vi "SOL Instruments LS.vi"() -> ()   [LabVIEW 2015]
doc: "Example VI that demonstrates all library features."
uses:
  PL SOL Instruments MS.lvclass
panel:
  in  "slit configuration":cluster{"width, um":dbl, "reset":bool}
  in  "slit":u8(ring)
  in  "mirror position index":u8(ring)
  in  "mirror":u8(ring)
  in  "shutter state":bool
  in  "shutter":u8(ring) items=["Shutter S1"]
  in  "turret configuration":T1 {"grating" items=["1200; 750", "1200; 280"]}
  in  "turret":u8(ring) items=["Change of the gratings"]
  in  "configuration file path":path
  out "SOL MS":refnum<class "PL SOL Instruments MS.lvclass">
  in  "port":refnum<visa-resource-name>
  out "error":errorcluster
  in  "stop":bool
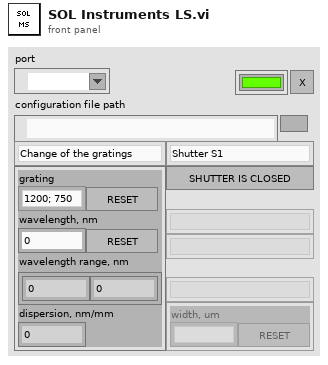
[diagram p1: front panel]
types:
  T1 = cluster{"grating":u8, "reset grating":bool, "wavelength, nm":dbl, "reset wavelength":bool, "wavelength range, nm":cluster{"min":dbl, "max":dbl}, "dispersion, nm/mm":dbl}
  T2 = cluster{"turrets":cluster{"name":string, "gratings":cluster{"name":string, "groove density, g/mm":dbl, "blaze wavelength, nm":dbl, "min wavelength, nm":dbl, "max wavelength, nm":dbl}[]}[], "shutters":cluster{"name":string}[], "mirrors":cluster{"name":string, "positions":cluster{"name":string}[]}[], "slits":cluster{"name":string, "min width, um":dbl, "max width, um":dbl}[]}
  T3 = cluster{"turrets":cluster{"current grating index":u8, "wavelength, nm":dbl, "dispersion, nm/mm":dbl}[], "shutters":cluster{"is open":bool}[], "mirrors":cluster{"current position index":u8}[], "slits":cluster{"width, um":dbl}[]}
  T4 = cluster{"name":string, "gratings":cluster{"name":string, "groove density, g/mm":dbl, "blaze wavelength, nm":dbl, "min wavelength, nm":dbl, "max wavelength, nm":dbl}[]}[]
  T5 = cluster{"current grating index":u8, "wavelength, nm":dbl, "dispersion, nm/mm":dbl}[]
  T6 = cluster{"name":string, "gratings":cluster{"name":string, "groove density, g/mm":dbl, "blaze wavelength, nm":dbl, "min wavelength, nm":dbl, "max wavelength, nm":dbl}[]}
  T7 = cluster{"current grating index":u8, "wavelength, nm":dbl, "dispersion, nm/mm":dbl}
  T8 = cluster{"name":string, "groove density, g/mm":dbl, "blaze wavelength, nm":dbl, "min wavelength, nm":dbl, "max wavelength, nm":dbl}[]
  T9 = cluster{"name":string, "groove density, g/mm":dbl, "blaze wavelength, nm":dbl, "min wavelength, nm":dbl, "max wavelength, nm":dbl}
  T10 = enum8{"Enabled", "Disabled", "Disabled and Grayed Out"}
  T11 = cluster{"name":string, "positions":cluster{"name":string}[]}[]
  T12 = cluster{"name":string, "min width, um":dbl, "max width, um":dbl}[]
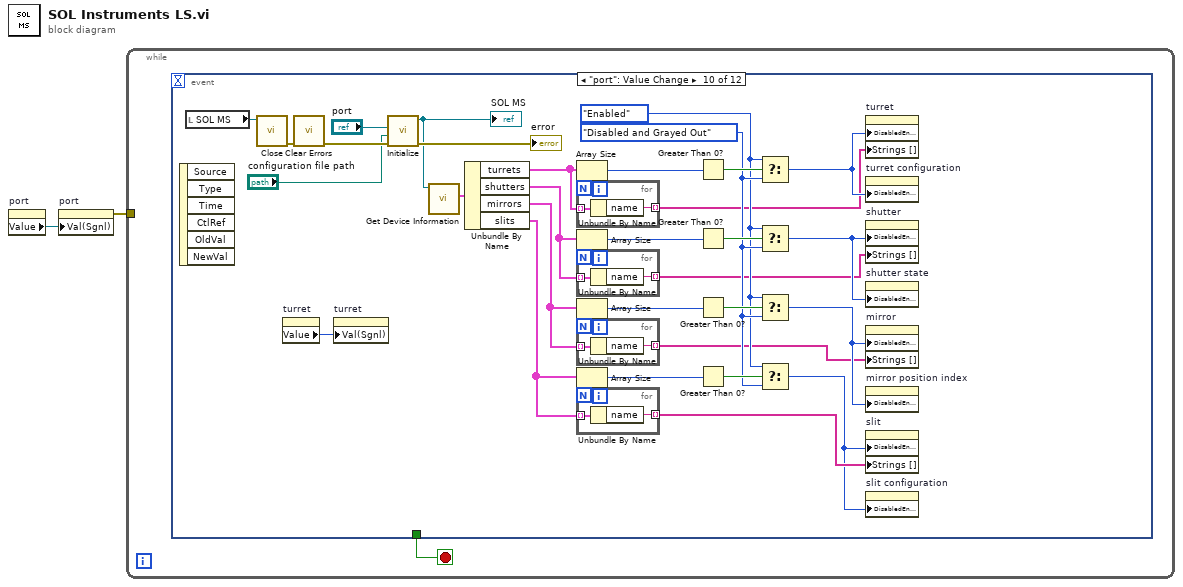
[diagram p0: block diagram]
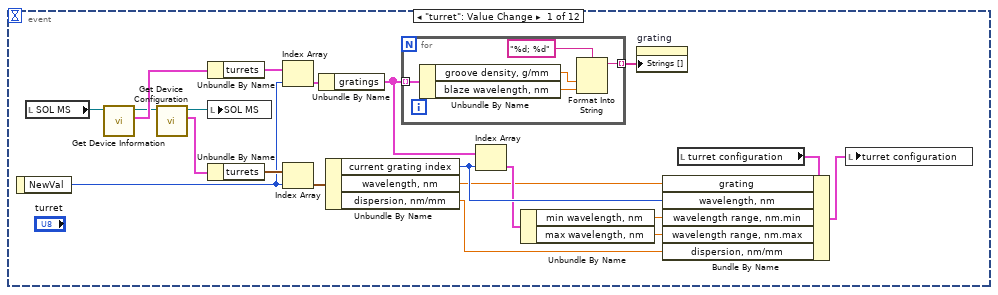
[diagram p2: hidden frame]
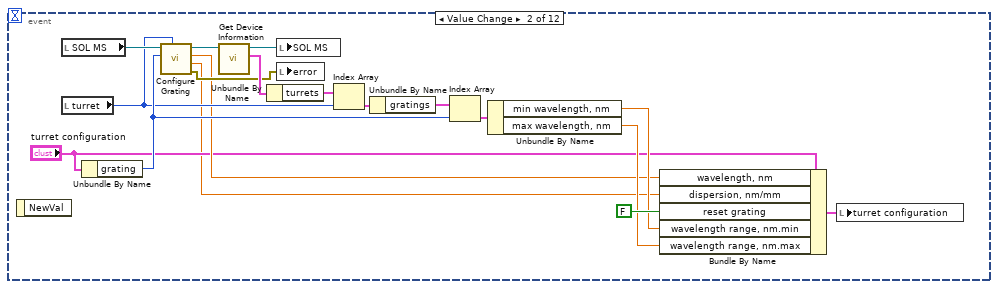
[diagram p3: hidden frame]
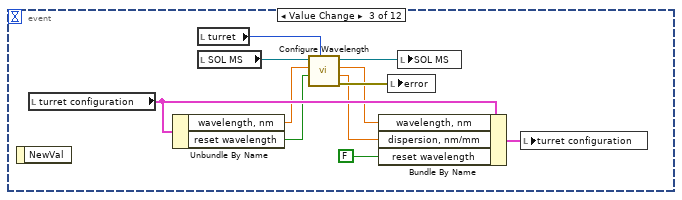
[diagram p4: hidden frame]
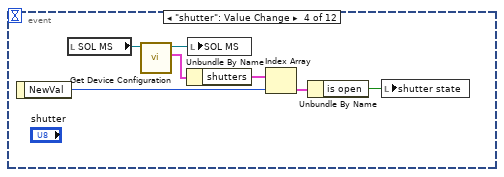
[diagram p5: hidden frame]
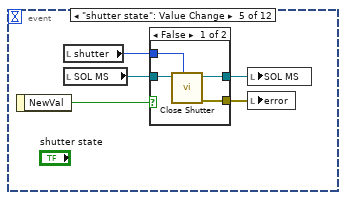
[diagram p6: hidden frame]
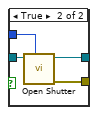
[diagram p7: hidden frame]
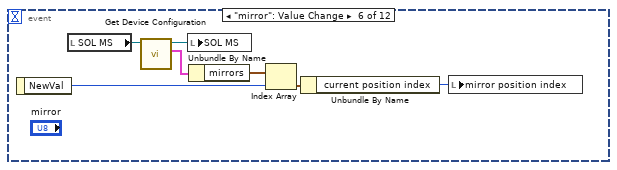
[diagram p8: hidden frame]
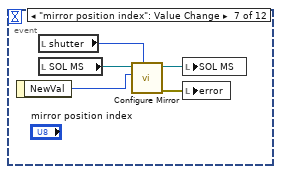
[diagram p9: hidden frame]
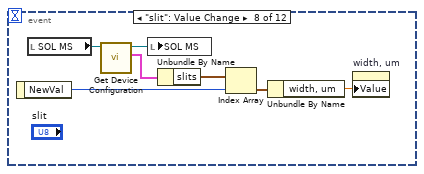
[diagram p10: hidden frame]
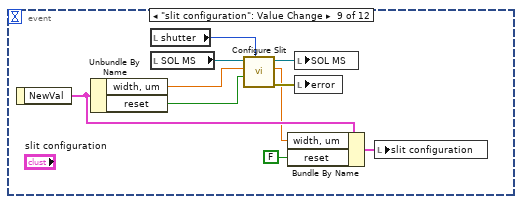
[diagram p11: hidden frame]
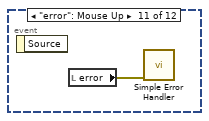
[diagram p12: hidden frame]
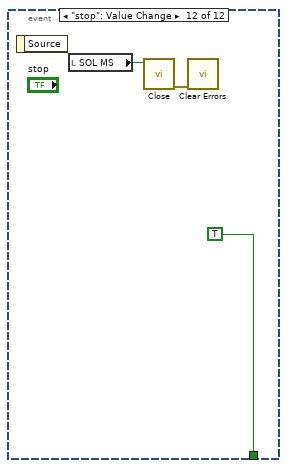
[diagram p13: hidden frame]
diagram:
  n1 = property on="port" class="VISAName"() -> ("Value"=w1:refnum<visa-resource-name>)  [unwired: 2 in, 2 out]
  n2 = property on="port" class="VISAName"("Val(Sgnl)"=w1) -> (error out=w2:errorcluster)  [unwired: 2 in, 1 out]
  n3 = while {
    tunnel: w2 -> [_]
    stop <- w3 stop-if-true
    n4 = event shown="[9] \"port\": Value Change" {
      selector: _ -> [_ _ _ _ _ _ _ _ _ _ _ _]
      dyn-events: _ -> [_ _ _ _ _ _ _ _ _ _ _ _]
      timeout: _ -> [_ _ _ _ _ _ _ _ _ _ _ _]
      tunnel: [_ _ _ _ _ _ _ _ _ _ _ TRUE ("stop")] -> w3
      event "turret": Value Change {
        n5 = event-data() -> ("NewVal"=w9:u8)  [unwired: 1 in]
        n6 = local read "SOL MS"() -> (w8:refnum<class "PL SOL Instruments MS.lvclass">)
        n7 = call "Get Device Information.vi"("SOL MS in"=w8) -> ("info"=w7:T2, "SOL MS out"=w6:refnum<class "PL SOL Instruments MS.lvclass">)  [unwired: 9 in]
        n8 = call "Get Device Configuration.vi"("SOL MS in"=w6) -> ("configuration"=w4:T3, "SOL MS out"=w5:refnum<class "PL SOL Instruments MS.lvclass">)  [unwired: 9 in]
        n9 = Unbundle By Name(w7) -> ("turrets"=w22:T4)
        n10 = local write "SOL MS"(w5) -> ()
        n11 = Unbundle By Name(w4) -> ("turrets"=w23:T5)
        n12 = Index Array(array=w22, index=w9) -> (element=w20:T6)
        n13 = Index Array(array=w23, index=w9) -> (element=w21:T7)
        n14 = Unbundle By Name(w20) -> ("gratings"=w16:T8)
        n15 = Unbundle By Name(w21) -> ("current grating index"=w15:u8, "wavelength, nm"=w13:dbl, "dispersion, nm/mm"=w10:dbl)
        n16 = for {
          tunnel: w16 -> [w28] mode=indexing
          tunnel: [w24] -> w17 mode=indexing
          n17 = Unbundle By Name(w28) -> ("groove density, g/mm"=w26:dbl, "blaze wavelength, nm"=w25:dbl)
          n18 = Format Into String(format string="%d; %d", w26, w25) -> (resulting string=w24:string)  [unwired: 2 in, 1 out]
        }
        n19 = Index Array(array=w16, index=w15) -> (element=w14:T9)
        n20 = Unbundle By Name(w14) -> ("min wavelength, nm"=w12:dbl, "max wavelength, nm"=w11:dbl)
        n21 = property on="grating" class="Ring (strict)"("Strings []"=w17) -> ()  [unwired: 2 in, 2 out]
        n22 = local read "turret configuration"() -> (w19:T1)
        n23 = Bundle By Name(cluster=w19, "grating"=w13, "wavelength, nm"=w15, "wavelength range, nm.min"=w12, "wavelength range, nm.max"=w11, "dispersion, nm/mm"=w10) -> (w18:T1)
        n24 = local write "turret configuration"(w18) -> ()
      }
      event "turret configuration.grating", "turret configuration.reset grating": Value Change {
        n25 = event-data() -> ()  [unwired: 1 in, 1 out]
        n26 = local read "SOL MS"() -> (w39:refnum<class "PL SOL Instruments MS.lvclass">)
        n27 = local read "turret"() -> (w37:u8)
        n28 = Unbundle By Name("turret configuration") -> ("grating"=w38:u8)
        n29 = call "Configure Grating.vi"("turret index (0)"=w37, "grating index"=w38, "SOL MS in"=w39) -> ("error out"=w33:errorcluster, "dispersion, nm/mm"=w30:dbl, "wavelength, nm"=w32:dbl, "SOL MS out"=w35:refnum<class "PL SOL Instruments MS.lvclass">)  [unwired: 5 in]
        n30 = call "Get Device Information.vi"("SOL MS in"=w35) -> ("info"=w34:T2, "SOL MS out"=w36:refnum<class "PL SOL Instruments MS.lvclass">)  [unwired: 9 in]
        n31 = Unbundle By Name(w34) -> ("turrets"=w45:T4)
        n32 = local write "SOL MS"(w36) -> ()
        n33 = local write "error"(w33) -> ()
        n34 = Index Array(array=w45, index=w37) -> (element=w44:T6)
        n35 = Unbundle By Name(w44) -> ("gratings"=w43:T8)
        n36 = Index Array(array=w43, index=w38) -> (element=w42:T9)
        n37 = Unbundle By Name(w42) -> ("min wavelength, nm"=w41:dbl, "max wavelength, nm"=w40:dbl)
        n38 = Bundle By Name(cluster="turret configuration", "wavelength, nm"=w32, "dispersion, nm/mm"=w30, "reset grating"=FALSE ("reset wavelength"), "wavelength range, nm.min"=w41, "wavelength range, nm.max"=w40) -> (w29:T1)
        n39 = local write "turret configuration"(w29) -> ()
      }
      event "turret configuration.wavelength, nm", "turret configuration.reset wavelength": Value Change {
        n40 = event-data() -> ()  [unwired: 1 in, 1 out]
        n41 = local read "turret configuration"() -> (w56:T1)
        n42 = Unbundle By Name(w56) -> ("wavelength, nm"=w52:dbl, "reset wavelength"=w51:bool)
        n43 = local read "turret"() -> (w53:u8)
        n44 = local read "SOL MS"() -> (w54:refnum<class "PL SOL Instruments MS.lvclass">)
        n45 = call "Configure Wavelength.vi"("turret index (0)"=w53, "reset (false)"=w51, "wavelength, nm"=w52, "SOL MS in"=w54) -> ("error out"=w50:errorcluster, "dispersion, nm/mm"=w47:dbl, "wavelength, nm"=w48:dbl, "SOL MS out"=w49:refnum<class "PL SOL Instruments MS.lvclass">)  [unwired: 4 in]
        n46 = Bundle By Name(cluster=w56, "wavelength, nm"=w48, "dispersion, nm/mm"=w47, "reset wavelength"=FALSE) -> (w55:T1)
        n47 = local write "error"(w50) -> ()
        n48 = local write "SOL MS"(w49) -> ()
        n49 = local write "turret configuration"(w55) -> ()
      }
      event "shutter": Value Change {
        n50 = event-data() -> ("NewVal"=w61:u8)  [unwired: 1 in]
        n51 = local read "SOL MS"() -> (w60:refnum<class "PL SOL Instruments MS.lvclass">)
        n52 = call "Get Device Configuration.vi"("SOL MS in"=w60) -> ("configuration"=w58:T3, "SOL MS out"=w59:refnum<class "PL SOL Instruments MS.lvclass">)  [unwired: 9 in]
        n53 = Unbundle By Name(w58) -> ("shutters"=w64:cluster{"is open":bool}[])
        n54 = local write "SOL MS"(w59) -> ()
        n55 = Index Array(array=w64, index=w61) -> (element=w63:cluster{"is open":bool})
        n56 = Unbundle By Name(w63) -> ("is open"=w62:bool)
        n57 = local write "shutter state"(w62) -> ()
      }
      event "shutter state": Value Change {
        n58 = event-data() -> ("NewVal"=w69:bool)  [unwired: 1 in]
        n59 = local read "shutter"() -> (w67:u8)
        n60 = local read "SOL MS"() -> (w68:refnum<class "PL SOL Instruments MS.lvclass">)
        n61 = case shown="False" w69 {
          tunnel: w68 -> [w73 w77]
          tunnel: w67 -> [w70 w76]
          tunnel: [w72 w75] -> w66
          tunnel: [w71 w74] -> w65
          frame False {
            n62 = call "Close Shutter.vi"("shutter index (0)"=w70, "SOL MS in"=w73) -> ("error out"=w71:errorcluster, "SOL MS out"=w72:refnum<class "PL SOL Instruments MS.lvclass">)  [unwired: 8 in]
          }
          frame True {
            n63 = call "Open Shutter.vi"("shutter index (0)"=w76, "SOL MS in"=w77) -> ("error out"=w74:errorcluster, "SOL MS out"=w75:refnum<class "PL SOL Instruments MS.lvclass">)  [unwired: 8 in]
          }
        }
        n64 = local write "SOL MS"(w66) -> ()
        n65 = local write "error"(w65) -> ()
      }
      event "mirror": Value Change {
        n66 = event-data() -> ("NewVal"=w81:u8)  [unwired: 1 in]
        n67 = local read "SOL MS"() -> (w80:refnum<class "PL SOL Instruments MS.lvclass">)
        n68 = call "Get Device Configuration.vi"("SOL MS in"=w80) -> ("configuration"=w78:T3, "SOL MS out"=w79:refnum<class "PL SOL Instruments MS.lvclass">)  [unwired: 9 in]
        n69 = local write "SOL MS"(w79) -> ()
        n70 = Unbundle By Name(w78) -> ("mirrors"=w84:cluster{"current position index":u8}[])
        n71 = Index Array(array=w84, index=w81) -> (element=w83:cluster{"current position index":u8})
        n72 = Unbundle By Name(w83) -> ("current position index"=w82:u8)
        n73 = local write "mirror position index"(w82) -> ()
      }
      event "mirror position index": Value Change {
        n74 = event-data() -> ("NewVal"=w85:u8)  [unwired: 1 in]
        n75 = local read "shutter"() -> (w86:u8)
        n76 = local read "SOL MS"() -> (w89:refnum<class "PL SOL Instruments MS.lvclass">)
        n77 = call "Configure Mirror.vi"("mirror index (0)"=w86, "mirror position index"=w85, "SOL MS in"=w89) -> ("error out"=w87:errorcluster, "SOL MS out"=w88:refnum<class "PL SOL Instruments MS.lvclass">)  [unwired: 7 in]
        n78 = local write "SOL MS"(w88) -> ()
        n79 = local write "error"(w87) -> ()
      }
      event "slit": Value Change {
        n80 = event-data() -> ("NewVal"=w94:u8)  [unwired: 1 in]
        n81 = local read "SOL MS"() -> (w93:refnum<class "PL SOL Instruments MS.lvclass">)
        n82 = call "Get Device Configuration.vi"("SOL MS in"=w93) -> ("configuration"=w91:T3, "SOL MS out"=w92:refnum<class "PL SOL Instruments MS.lvclass">)  [unwired: 9 in]
        n83 = local write "SOL MS"(w92) -> ()
        n84 = Unbundle By Name(w91) -> ("slits"=w96:cluster{"width, um":dbl}[])
        n85 = Index Array(array=w96, index=w94) -> (element=w95:cluster{"width, um":dbl})
        n86 = Unbundle By Name(w95) -> ("width, um"=w90:dbl)
        n87 = property on="width, um" class="Ring (strict)"("Value"=w90) -> ()  [unwired: 2 in, 2 out]
      }
      event "slit configuration": Value Change {
        n88 = event-data() -> ("NewVal"=w100:cluster{"width, um":dbl, "reset":bool})  [unwired: 1 in]
        n89 = Unbundle By Name(w100) -> ("width, um"=w102:dbl, "reset"=w101:bool)
        n90 = local read "shutter"() -> (w106:u8)
        n91 = local read "SOL MS"() -> (w103:refnum<class "PL SOL Instruments MS.lvclass">)
        n92 = call "Configure Slit.vi"("slit index (0)"=w106, "reset (false)"=w101, "width, um"=w102, "SOL MS in"=w103) -> ("error out"=w104:errorcluster, "width, um"=w98:dbl, "SOL MS out"=w105:refnum<class "PL SOL Instruments MS.lvclass">)  [unwired: 5 in]
        n93 = Bundle By Name(cluster=w100, "width, um"=w98, "reset"=FALSE) -> (w99:cluster{"width, um":dbl, "reset":bool})
        n94 = local write "SOL MS"(w105) -> ()
        n95 = local write "error"(w104) -> ()
        n96 = local write "slit configuration"(w99) -> ()
      }
      event "port": Value Change {
        w117 = T10."Disabled and Grayed Out" ("Disabled")
        w116 = T10."Enabled" ("Disabled")
        n97 = event-data() -> ()  [unwired: 1 in, 6 out]
        n98 = local read "SOL MS"() -> (w137:refnum<class "PL SOL Instruments MS.lvclass">)
        n99 = call "Close.vi"("Comdel in"=w137) -> ("error out"=w135:errorcluster)  [unwired: 10 in]
        n100 = property on="turret" class="Ring (strict)"() -> ("Value"=w107:u8)  [unwired: 2 in, 2 out]
        n101 = call <vilib>:"Clear Errors.vi"("error in (no error)"=w135) -> ("error out"=w136:errorcluster)  [unwired: 5 in, 1 out]
        n102 = property on="turret" class="Ring (strict)"("Val(Sgnl)"=w107) -> ()  [unwired: 2 in, 2 out]
        n103 = call "Initialize.vi"("error in (no error)"=w136, "configuration file path"="configuration file path", "port"="port") -> ("error out"=→"error":errorcluster, "SOL MS out"=w131:refnum<class "PL SOL Instruments MS.lvclass">)  [unwired: 7 in]
        "SOL MS" <- w131
        n104 = call "Get Device Information.vi"("SOL MS in"=w131) -> ("info"=w130:T2)  [unwired: 9 in, 1 out]
        n105 = Unbundle By Name(w130) -> ("turrets"=w126:T4, "shutters"=w127:cluster{"name":string}[], "mirrors"=w128:T11, "slits"=w129:T12)
        n106 = Array Size(array=w126) -> (size(s)=w125:i32)
        n107 = for {
          tunnel: w126 -> [w145] mode=indexing
          tunnel: [w144] -> w114 mode=indexing
          n108 = Unbundle By Name(w145) -> ("name"=w144:string)
        }
        n109 = Array Size(array=w127) -> (size(s)=w123:i32)
        n110 = for {
          tunnel: w127 -> [w143] mode=indexing
          tunnel: [w142] -> w112 mode=indexing
          n111 = Unbundle By Name(w143) -> ("name"=w142:string)
        }
        n112 = Array Size(array=w128) -> (size(s)=w121:i32)
        n113 = for {
          tunnel: w128 -> [w141] mode=indexing
          tunnel: [w140] -> w110 mode=indexing
          n114 = Unbundle By Name(w141) -> ("name"=w140:string)
        }
        n115 = Array Size(array=w129) -> (size(s)=w118:i32)
        n116 = for {
          tunnel: w129 -> [w139] mode=indexing
          tunnel: [w138] -> w109 mode=indexing
          n117 = Unbundle By Name(w139) -> ("name"=w138:string)
        }
        n118 = Greater Than 0?(x=w125) -> (x > 0?=w124:bool)
        n119 = Greater Than 0?(x=w123) -> (x > 0?=w122:bool)
        n120 = Greater Than 0?(x=w121) -> (x > 0?=w120:bool)
        n121 = Greater Than 0?(x=w118) -> (x > 0?=w119:bool)
        n122 = Select(t=w116, s=w124, f=w117) -> (s? t:f=w115:T10)
        n123 = Select(t=w116, s=w122, f=w117) -> (s? t:f=w113:T10)
        n124 = Select(t=w116, s=w120, f=w117) -> (s? t:f=w111:T10)
        n125 = Select(t=w116, s=w119, f=w117) -> (s? t:f=w108:T10)
        n126 = property on="turret" class="Ring (strict)"("DisabledEnum"=w115, "Strings []"=w114) -> ()  [unwired: 2 in, 2 out]
        n127 = property on="turret configuration" class="Clust (strict)"("DisabledEnum"=w115) -> ()  [unwired: 2 in, 2 out]
        n128 = property on="shutter" class="Ring (strict)"("DisabledEnum"=w113, "Strings []"=w112) -> ()  [unwired: 2 in, 2 out]
        n129 = property on="shutter state" class="Bool (strict)"("DisabledEnum"=w113) -> ()  [unwired: 2 in, 2 out]
        n130 = property on="mirror" class="Ring (strict)"("DisabledEnum"=w111, "Strings []"=w110) -> ()  [unwired: 2 in, 2 out]
        n131 = property on="mirror position index" class="Ring (strict)"("DisabledEnum"=w111) -> ()  [unwired: 2 in, 2 out]
        n132 = property on="slit" class="Ring (strict)"("DisabledEnum"=w108, "Strings []"=w109) -> ()  [unwired: 2 in, 2 out]
        n133 = property on="slit configuration" class="Clust (strict)"("DisabledEnum"=w108) -> ()  [unwired: 2 in, 2 out]
      }
      event "error": Mouse Up {
        n134 = event-data() -> ()  [unwired: 1 in, 1 out]
        n135 = local read "error"() -> (w146:errorcluster)
        n136 = call <vilib>:"Simple Error Handler.vi"("error in (no error)"=w146) -> ()  [unwired: 4 in, 5 out]
      }
      event "stop": Value Change {
        n137 = event-data() -> ()  [unwired: 1 in, 1 out]
        n138 = local read "SOL MS"() -> (w148:refnum<class "PL SOL Instruments MS.lvclass">)
        n139 = call "Close.vi"("Comdel in"=w148) -> ("error out"=w147:errorcluster)  [unwired: 10 in]
        n140 = call <vilib>:"Clear Errors.vi"("error in (no error)"=w147) -> ()  [unwired: 5 in, 2 out]
      }
    }
  }
